vi "Delete Uint64 DVR.vi"(8 "error in (no error)":errorcluster, 11 "Uint64 DVR in":refnum<data-value>) -> (0 "error out":errorcluster, 3 "Uint64 out":refnum<class "Uint64.lvclass">)   [LabVIEW 2015, in "MDSplus.lvlib" / "Uint64.lvclass"]
uses:
  <vilib>/MDSplus/Classes/Data_Class/Scalar_Class/Uint64_Class/Uint64.lvclass
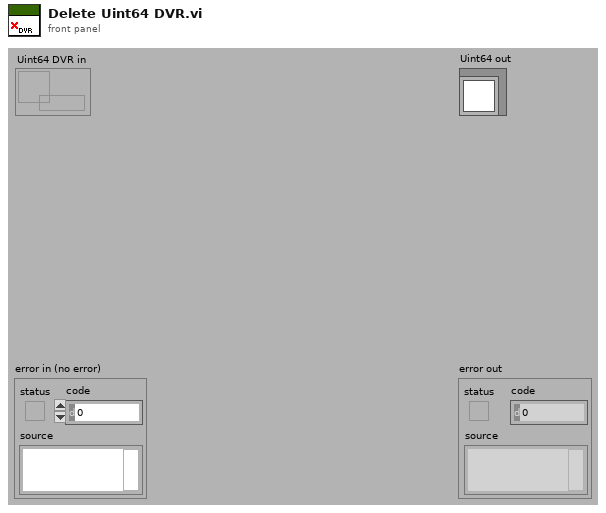
[diagram p1: front panel]
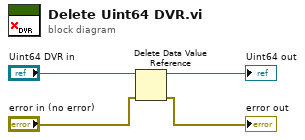
[diagram p0: block diagram]
diagram:
  n1 = Delete Data Value Reference(data value reference="Uint64 DVR in", error in="error in (no error)") -> (data value=→"Uint64 out":refnum<class "Uint64.lvclass">, error out=→"error out":errorcluster)
